vi "LV8_9.vi"() -> ()   [LabVIEW 2016]
uses:
  <vilib>/imath/engines/lvmath2/RunTimeEngine/RangeToken/NIMS_Range.vi
  <instcachedir>/0/NIMS_Range_A7C094595B484CA7AF10685B02D808ED.lvgen/NIMS_Range_A7C094595B484CA7AF10685B02D808ED_000.vi
  <vilib>/imathl/engines/lvmath/Functions/Error Handling/Create Error.vi
  <vilib>/imath/engines/lvmath2/RunTimeEngine/ArithmeticOperatorToken/NIMS_ArithmeticOperator_plus.vi
  <instcachedir>/0/NIMS_ArithmeticOperator_plus_0120E0498A0F4B4B9BDCAC2554767A4E.lvgen/NIMS_ArithmeticOperator_plus_0120E0498A0F4B4B9BDCAC2554767A4E_004.vi
  <vilib>/imath/engines/lvmath2/RunTimeEngine/BuiltInFunctions/fft/NIMS_fft(GV).vi
  <instcachedir>/0/NIMS_fft(GV)_4C6467FC22F84E4BA42517A07EF978B0.lvgen/NIMS_fft(GV)_4C6467FC22F84E4BA42517A07EF978B0_000.vi
  <vilib>/imath/engines/lvmath2/RunTimeEngine/ErrorHandling/NIMS_Error From Error Code.vi
  <vilib>/imath/engines/lvmath2/RunTimeEngine/BuiltInFunctions/abs/NIMS_abs(signed).vi
  <instcachedir>/0/NIMS_abs(signed)_C4FCB8E6058B49B797C7C8D53CA5F6EC.lvgen/NIMS_abs(signed)_C4FCB8E6058B49B797C7C8D53CA5F6EC_006.vi
  <vilib>/imath/engines/lvmath2/RunTimeEngine/BuiltInFunctions/fftshift/NIMS_fftshift(GV).vi
  <instcachedir>/0/NIMS_fftshift(GV)_BD7A7BA9CA6B470B9A9F73A6A3FEEB3E.lvgen/NIMS_fftshift(GV)_BD7A7BA9CA6B470B9A9F73A6A3FEEB3E_001.vi
  <vilib>/imath/engines/lvmath2/RunTimeEngine/NodeEndStatement/NIMS_NodeEndStatement_Output.vi
  <instcachedir>/0/NIMS_NodeEndStatement_Output_53EC0D466D134D7ABD903AC30B43404B.lvgen/NIMS_NodeEndStatement_Output_53EC0D466D134D7ABD903AC30B43404B_005.vi
  <vilib>/imath/engines/lvmath2/RunTimeEngine/ErrorHandling/NIMS_Finalize Error.vi
panel:
  in  "stop":bool
  in  "Amplitude 2 @ 10 Hz":dbl(slide)=10.0 scale=0.0..10.0
  in  "Amplitude 1 @ 5 Hz":dbl(slide)=4.0 scale=0.0..10.0
  in  "dc":dbl(slide)=1.0 scale=0.0..10.0
  out "time domain":cluster{"f":dbl[], "FXX":dbl[]}(graph)={"f"=[0.0, 0.02, 0.04, 0.06, 0.08, 0.1, 0.12, 0.14, 0.16, 0.18], "FXX"=[9.000006652754788, 0.1169483584169746, -5.194621571904596, 1.8587910278832935, 11.529609681550545, 9.000006652754793, -4.585333659922803, -12.803073702265825, -5.749661102477939, 6.827327663210756]}
  out "frequency domain":cluster{"f":dbl[], "FXX":dbl[]}(graph)={"f"=[-25.0, -20.0, -15.0, -10.0, -5.0, 0.0, 5.0, 10.0, 15.0, 20.0], "FXX"=[2.6645352591003756e-16, 5.693865149565923e-16, 5.944986251656775e-16, 4.999999999999999, 2.0000000000000004, 0.9999999999999986, 2.0000000000000004, 4.999999999999999, 5.944986251656775e-16, 5.693865149565923e-16]}
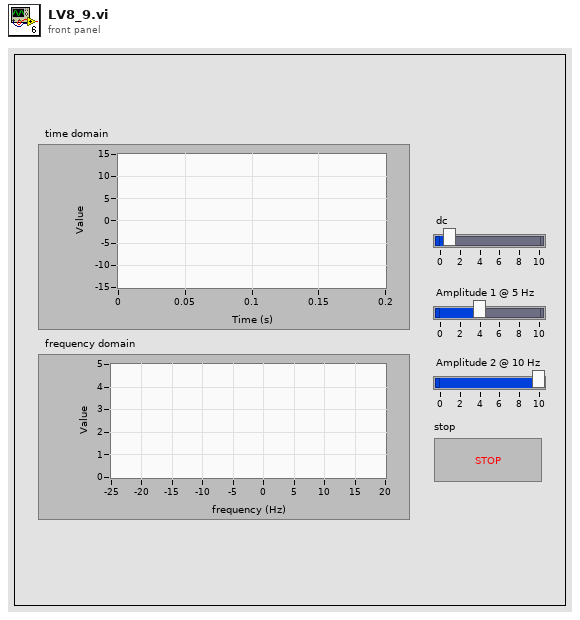
[diagram p1: front panel]
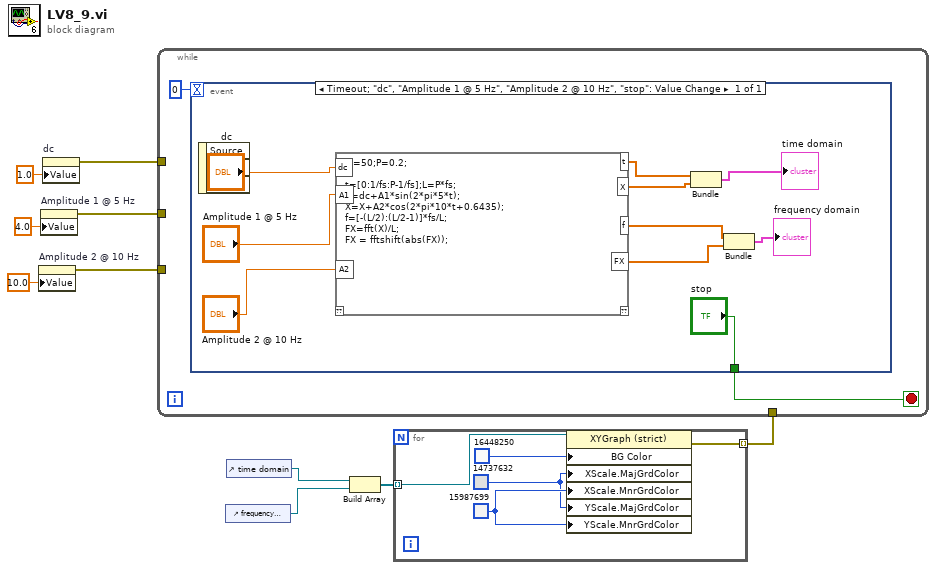
[diagram p0: block diagram]
diagram:
  n1 = property on="Amplitude 2 @ 10 Hz" class="Slide (strict)"("Value"=10.0 ("Amplitude 2 @ 10 Hz")) -> (error out=w8:errorcluster)  [unwired: 2 in, 1 out]
  n2 = property on="Amplitude 1 @ 5 Hz" class="Slide (strict)"("Value"=4.0 ("Amplitude 1 @ 5 Hz")) -> (error out=w9:errorcluster)  [unwired: 2 in, 1 out]
  n3 = property on="dc" class="Slide (strict)"("Value"=1.0 ("dc")) -> (error out=w10:errorcluster)  [unwired: 2 in, 1 out]
  n4 = control-ref of="frequency domain"() -> (w2:refnum<vi>)
  n5 = control-ref of="time domain"() -> (w3:refnum<vi>)
  n6 = Build Array(w3, w2) -> (w4:refnum<vi>[])
  n7 = for {
    tunnel: w4 -> [w12] mode=indexing
    tunnel: [w11] -> w1 mode=indexing
    w14 = u32 15987699
    w13 = u32 14737632
    n8 = property class="XYGraph (strict)"(reference=w12, "BG Color"=u32 16448250, "XScale.MajGrdColor"=w13, "XScale.MnrGrdColor"=w14, "YScale.MajGrdColor"=w13, "YScale.MnrGrdColor"=w14) -> (error out=w11:errorcluster)  [unwired: 1 in, 1 out]
  }
  n9 = while {
    tunnel: w10 -> [_]
    tunnel: w9 -> [_]
    tunnel: w8 -> [_]
    tunnel: w1 -> [_]
    stop <- w17 stop-if-true
    n10 = event shown="[0] Timeout;  \"dc\", \"Amplitude 1 @ 5 Hz\", \"Amplitude 2 @ 10 Hz\", \"stop\": Value Change" {
      selector: _ -> [_]
      dyn-events: _ -> [_]
      timeout: 0 -> [_]
      tunnel: ["stop"] -> w17
      event Timeout; "dc", "Amplitude 1 @ 5 Hz", "Amplitude 2 @ 10 Hz", "stop": Value Change {
        n11 = event-data() -> ()  [unwired: 1 in, 3 out]
        n12 = mathscript code="fs=50;P=0.2;\n\nt=[0:1/fs:P-1/fs];L=P*fs;\nX=dc+A1*sin(2*pi*5*t);\nX=X+A2*cos(2*pi*10*t+0.6435);\nf=[-(L/2):(L/2-1)]*fs/L;\nFX=fft(X)/L;\nFX = fftshift(abs(FX));"("dc"="dc", "A1"="Amplitude 1 @ 5 Hz", "A2"="Amplitude 2 @ 10 Hz") -> ("f"=w27:dbl[], "FX"=w26:dbl[], "X"=w23:dbl[], "t"=w24:dbl[])  [unwired: 1 in, 1 out]
        n13 = Bundle("t"=w24, "X"=w23) -> (→"time domain":cluster{"t":dbl[], "X":dbl[]})  [unwired: 1 in]
        n14 = Bundle("f"=w27, "FX"=w26) -> (→"frequency domain":cluster{"f":dbl[], "FX":dbl[]})  [unwired: 1 in]
      }
    }
  }
